vi "Set Switcher Monitor Card2023.vi"(0 "Device Configuration":T1={"Relay Type"=0, "GPIB Address"=6, "GPIB Card"=0} {"GPIB Card" min=0 max=30; "GPIB Address" min=0 max=30; "Relay Type" items=["HP3488A (44472A)", "HP34970A (34905A)"]}, 1 "Slot (Card)":i8=1 min=0 max=5, 2 "Group":i8=1 min=0 max=2, 3 "Channel":i8=1 min=0 max=4) -> (4 "Command Failed":bool)   [LabVIEW 2023]
doc: "Changes the display on the switcher to indicate closed positions for a particular slot (card).\n\nIf a '0' is connected to Slot (Card), monitoring mode will be turned off (closed positions will not show up on the display).\n\nCurrently supports:\n\nHP3488A (44472A)"
panel:
  # "Configuration"
  # "Settings"
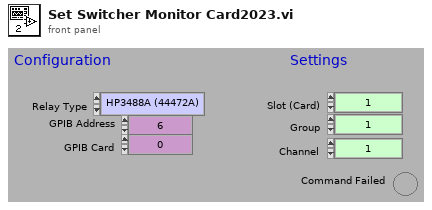
[diagram p1: front panel]
types:
  T1 = cluster{"Relay Type":i8, "GPIB Address":i8, "GPIB Card":i8}
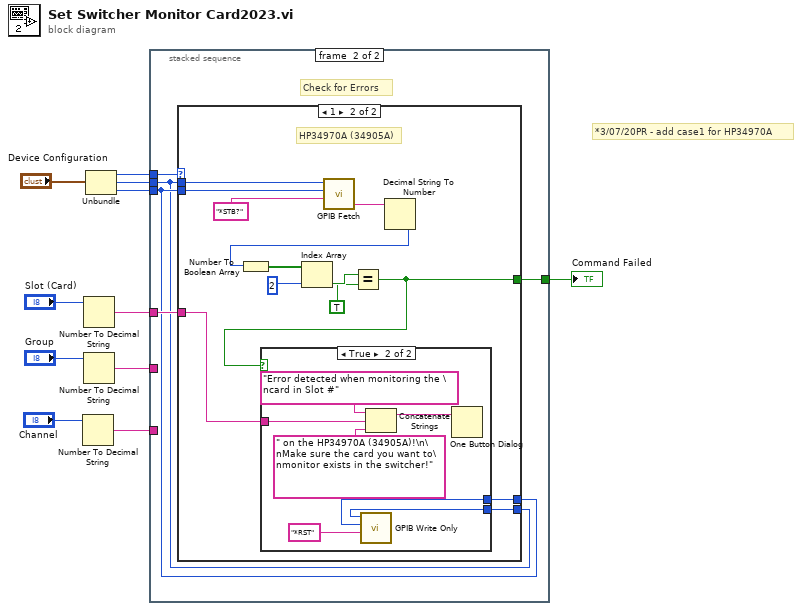
[diagram p0: block diagram]
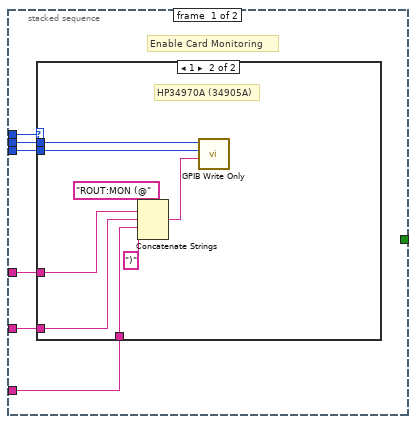
[diagram p2: hidden frame]
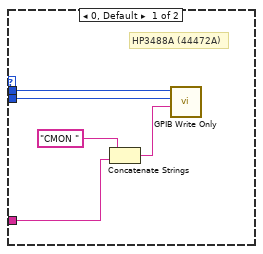
[diagram p3: hidden frame]
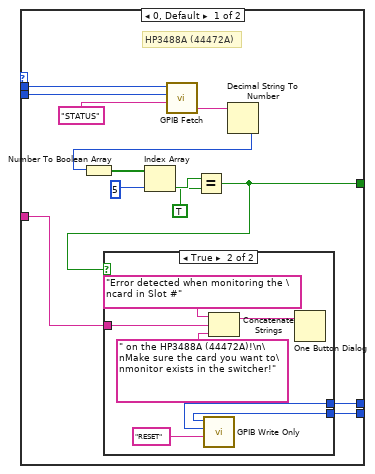
[diagram p4: hidden frame]
diagram:
  # "*3/07/20PR - add case1 for HP34970A"
  n1 = Number To Decimal String(number="Channel") -> (decimal integer string=w1:string)  [unwired: 1 in]
  n2 = Number To Decimal String(number="Slot (Card)") -> (decimal integer string=w8:string)  [unwired: 1 in]
  n3 = Number To Decimal String(number="Group") -> (decimal integer string=w2:string)  [unwired: 1 in]
  n4 = Unbundle("Device Configuration") -> ("Relay Type"=w10:i8, "GPIB Address"=w6:i8, "GPIB Card"=w5:i8)
  n5 = stacked-sequence {
    tunnel: w5 -> [w17 w32]
    tunnel: w6 -> [w16 w31]
    tunnel: w10 -> [w15 w35]
    tunnel: w8 -> [w14 w34]
    tunnel: [_ w33] -> w7
    tunnel: w2 -> [w13 _]
    tunnel: w1 -> [w12 _]
    frame #0 {
      # "Enable Card Monitoring"
      n6 = case shown="1" w15 {
        tunnel: w16 -> [w22 w30]
        tunnel: w17 -> [w21 w29]
        tunnel: w14 -> [w18 w26]
        tunnel: w13 -> [_ w25]
        tunnel: w12 -> [_ w24]
        frame 0, Default {
          # "HP3488A (44472A)"
          n7 = Concatenate Strings("CMON ", w18) -> (w19:string)
          n8 = call "GPIB Write Only.vi"("Command String"=w19, "GPIB Card"=w21, "GPIB Address"=w22) -> ()  [unwired: 3 in, 1 out]
        }
        frame 1 {
          # "HP34970A (34905A)"
          n9 = Concatenate Strings("ROUT:MON (@", w26, w25, w24, ")" ("string")) -> (w27:string)
          n10 = call "GPIB Write Only.vi"("Command String"=w27, "GPIB Card"=w29, "GPIB Address"=w30) -> ()  [unwired: 3 in, 1 out]
        }
      }
    }
    frame #1 {
      # "Check for Errors"
      n11 = case shown="1" w35 {
        tunnel: w31 -> [w41 w61]
        tunnel: w32 -> [w48 w68]
        tunnel: w34 -> [w40 w60]
        tunnel: [w38 w58] -> w33
        tunnel: w31 -> [w37 w57]
        tunnel: w32 -> [w36 w56]
        frame 0, Default {
          # "HP3488A (44472A)"
          n12 = call "GPIB Fetch.vi"("Command String"="STATUS", "GPIB Card"=w48, "GPIB Address"=w41) -> ("Characters Read"=w42:string)  [unwired: 1 in, 2 out]
          n13 = Decimal String To Number(string=w42) -> (number=w43:i32)  [unwired: 2 in, 1 out]
          n14 = Number To Boolean Array(number=w43) -> (Boolean array=w44:bool[])
          n15 = Index Array(array=w44, index=5) -> (element=w47:bool)
          n16 = Equal?(x=w47, y=TRUE) -> (x = y?=w38:bool)
          n17 = case shown="True" w38 {
            tunnel: w40 -> [_ w52]
            tunnel: w37 -> [_ w50]
            tunnel: w36 -> [_ w49]
            frame False {
            }
            frame True {
              n18 = call "GPIB Write Only.vi"("Command String"="RESET", "GPIB Card"=w49, "GPIB Address"=w50) -> ()  [unwired: 3 in, 1 out]
              n19 = Concatenate Strings("Error detected when monitoring the \ncard in Slot #", w52, " on the HP3488A (44472A)!\n\nMake sure the card you want to\nmonitor exists in the switcher!") -> (w54:string)
              n20 = One Button Dialog(message=w54) -> ()  [unwired: 1 in, 1 out]
            }
          }
        }
        frame 1 {
          # "HP34970A (34905A)"
          n21 = call "GPIB Fetch.vi"("Command String"="*STB?", "GPIB Card"=w68, "GPIB Address"=w61) -> ("Characters Read"=w62:string)  [unwired: 1 in, 2 out]
          n22 = Decimal String To Number(string=w62) -> (number=w63:i32)  [unwired: 2 in, 1 out]
          n23 = Number To Boolean Array(number=w63) -> (Boolean array=w64:bool[])
          n24 = Index Array(array=w64, index=2) -> (element=w67:bool)
          n25 = Equal?(x=w67, y=TRUE) -> (x = y?=w58:bool)
          n26 = case shown="True" w58 {
            tunnel: w60 -> [_ w72]
            tunnel: w57 -> [_ w70]
            tunnel: w56 -> [_ w69]
            frame False {
            }
            frame True {
              n27 = call "GPIB Write Only.vi"("Command String"="*RST", "GPIB Card"=w69, "GPIB Address"=w70) -> ()  [unwired: 3 in, 1 out]
              n28 = Concatenate Strings("Error detected when monitoring the \ncard in Slot #", w72, " on the HP34970A (34905A)!\n\nMake sure the card you want to\nmonitor exists in the switcher!") -> (w74:string)
              n29 = One Button Dialog(message=w74) -> ()  [unwired: 1 in, 1 out]
            }
          }
        }
      }
    }
  }
  "Command Failed" <- w7
